vi "set_destination.vi"(0 "HGF_Agent in":refnum<class "MoAgSy_AgentBase.lvclass">, 2 "destination":string, 5 "error in (no error)":errorcluster) -> (14 "HGF_Agent out":refnum<class "MoAgSy_AgentBase.lvclass">, 19 "error out":errorcluster)   [LabVIEW 2009, in "MoAgSy_Base.lvlib" / "MoAgSy_AgentBase.lvclass"]
uses:
  MoAgSy_AgentBase.lvclass
  MoAgSy_AgentBase.lvclass/MoAgSy_AgentBase.ctl
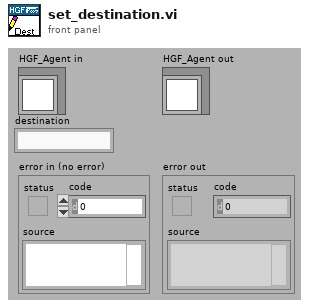
[diagram p1: front panel]
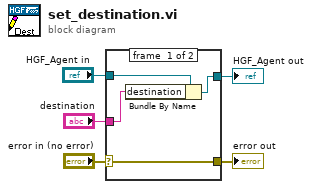
[diagram p0: block diagram]
diagram:
  n1 = case shown="No Error" "error in (no error)" {
    selector: "error in (no error)" -> [w9 w11]
    tunnel: [w9 w11] -> w4
    tunnel: [w7 w10] -> w2
    tunnel: "HGF_Agent in" -> [w8 w10]
    tunnel: "destination" -> [w6 _]
    frame #0 {
      n2 = Bundle By Name(cluster=w8, "destination"=w6) -> (w7:refnum<class "MoAgSy_AgentBase.lvclass">)
    }
    frame #1 {
    }
  }
  "error out" <- w4
  "HGF_Agent out" <- w2
